vi "Stop Core.vi"(10 "final error code":i32, 11 "Command Handler in":refnum<class "Command Handler.lvclass">) -> (3 "Command Handler out":refnum<class "Command Handler.lvclass">)   [LabVIEW 2015, in "Command Handler.lvlib" / "Command Handler.lvclass"]
doc: "(<B>Filename</B>: Actor Framework.lvlib:Actor.lvclass:Stop Core.vi)\n\nDefines what the actor does before it stops. Use the <B>final error code</B> input to determine whether the actor shut down in response to an error.\n\nBy default, this method does nothing. A descendant class may override it to define behavior, such as shutting down any processes the actor initiated in its override of the Actor Core method."
uses:
  Command Handler.lvclass
  <vilib>/ActorFramework/Actor/Actor.lvclass
  Command Handler.lvlib
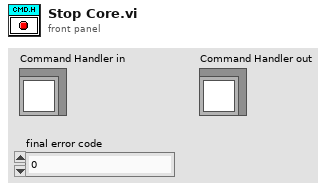
[diagram p1: front panel]
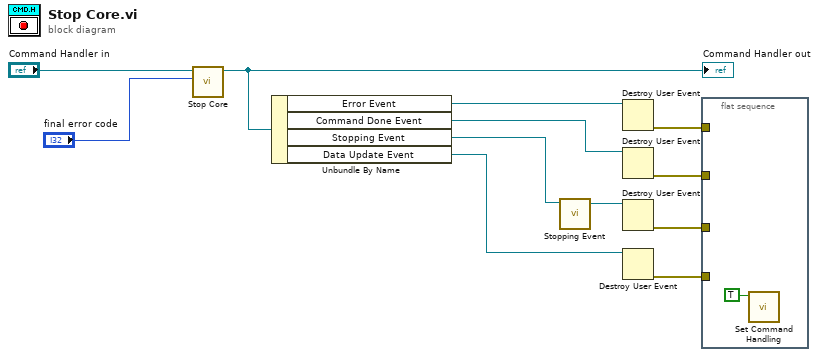
[diagram p0: block diagram]
diagram:
  n1 = call-parent "Stop Core.vi"("final error code"="final error code", "Actor in"="Command Handler in") -> ("Actor out"=w10:refnum<class "Command Handler.lvclass">)  [unwired: 9 in]
  "Command Handler out" <- w10
  n2 = Unbundle By Name(w10) -> ("Error Event"=w9:refnum<user-event>, "Command Done Event"=w3:refnum<user-event>, "Stopping Event"=w5:refnum<user-event>, "Data Update Event"=w2:refnum<user-event>)
  n3 = call "Stopping Event.vi"("User Event in"=w5) -> ("User Event out"=w4:refnum<user-event>)  [unwired: 10 in]
  n4 = Destroy User Event(user event=w9) -> (error out=w8:errorcluster)  [unwired: 1 in]
  n5 = Destroy User Event(user event=w3) -> (error out=w7:errorcluster)  [unwired: 1 in]
  n6 = Destroy User Event(user event=w4) -> (error out=w6:errorcluster)  [unwired: 1 in]
  n7 = Destroy User Event(user event=w2) -> (error out=w1:errorcluster)  [unwired: 1 in]
  n8 = flat-sequence {
    tunnel: w8 -> [_]
    tunnel: w7 -> [_]
    tunnel: w6 -> [_]
    tunnel: w1 -> [_]
    frame #0 {
      n9 = call "Set Command Handling.vi"("Disable Command Handling"=TRUE ("Command Handling Stopped")) -> ()  [unwired: 10 in, 1 out]
    }
  }
